vi "After Launch Init.vi"(8 "error in (no error)":errorcluster, 11 "LS218 in":refnum<class "LS218.lvclass">) -> (0 "error out":errorcluster, 3 "LS218 out":refnum<class "LS218.lvclass">)   [LabVIEW 2013, in "LS218.lvlib" / "LS218.lvclass"]
doc: "Use <b>Pre Launch init.vi</b> method for sanity checks that are supposed to prevent the actor from launching if they fail. Use <B>this</B> method instead to initialize this actor when it has been activated. A corresponding high priority message will become dispatched before the <B>Actor Core.vi</b> is called.\n\n<b>Derived classed should call the parent methode first</b> and their own initialization code after.\n\nRefer also to the ongoing discussion at https://decibel.ni.com/content/message/57394#57394."
uses:
  LS218.lvclass
  LS218 Messages/Read All Sensor Data Msg/Read All Sensor Data Msg.lvclass
  LS218.lvclass/LS218.ctl
  CSPP_Core/Classes/CS++ProcessVariables/PVConnection/PVConnection.lvclass
  CSPP_Core/Actors/CS++DeviceActor/CS++DeviceActor.lvclass
  <vilib>/ActorFramework/Actor/Actor.lvclass/Actor.ctl
  <vilib>/ActorFramework/Message Enqueuer/Message Enqueuer.lvclass/Message Enqueuer.ctl
  CSPP_Core/Actors/CS++DeviceActor/CS++DeviceActor.lvclass/CS++DeviceActor.ctl
  <vilib>/ActorFramework/Message Enqueuer/Init from Existing Queue.vi
  <vilib>/ActorFramework/Message Enqueuer/Enqueue.vi
  <vilib>/ActorFramework/Message Priority Queue/Priority Enqueue.vi
  <vilib>/ActorFramework/Message Enqueuer/Message Enqueuer.lvclass
  LS218 Messages/Write calibration curves to instruments Msg/Write calibration curves to instruments Msg.lvclass
  <vilib>/ActorFramework/Actor/Actor.lvclass
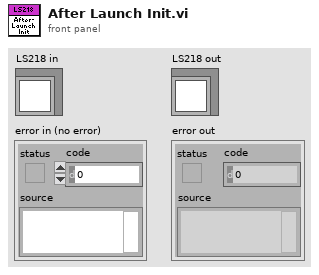
[diagram p1: front panel]
types:
  T1 = cluster{"Write Access":enum8{"Allowed", "Required", "None"}, "Read Access":enum8{"Allowed", "Required", "None"}}
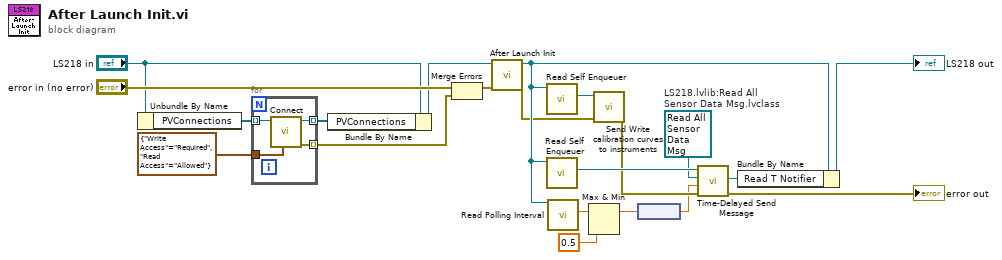
[diagram p0: block diagram]
diagram:
  w3 = refnum<class "Read All Sensor Data Msg.lvclass"> refnum  # LS218.lvlib:Read All Sensor Data Msg.lvclass
  n1 = Unbundle By Name("LS218 in") -> ("PVConnections"=w19:refnum<class "PVConnection.lvclass">[])
  n2 = for {
    tunnel: w19 -> [w25] mode=indexing
    tunnel: [w24] -> w18 mode=indexing
    tunnel: T1 {"Write Access"=enum."Required", "Read Access"=enum."Allowed"} ("Access") -> [w23]
    tunnel: [w22] -> w13 mode=indexing
    n3 = call-dynamic "Connect.vi"("Access (R/W allowed)"=w23, "PVConnection in"=w25) -> ("error out"=w22:errorcluster, "PVConnection out"=w24:refnum<class "PVConnection.lvclass">)  [unwired: 8 in]
  }
  n4 = Bundle By Name(cluster="LS218 in", "PVConnections"=w18) -> (w15:refnum<class "LS218.lvclass">)
  n5 = Merge Errors("error in (no error)", w13) -> (w14:errorcluster)
  n6 = call-parent "After Launch Init.vi"("error in (no error)"=w14, "CS++DeviceActor in"=w15) -> ("error out"=w1:errorcluster, "CS++DeviceActor out"=w2:refnum<class "LS218.lvclass">)  [unwired: 8 in]
  n7 = call <vilib>:"Read Self Enqueuer.vi"("Actor"=w2) -> ("Self Enqueuer"=w20:refnum<class "Message Enqueuer.lvclass">)  [unwired: 10 in]
  n8 = call <vilib>:"Read Self Enqueuer.vi"("Actor"=w2) -> ("Self Enqueuer"=w12:refnum<class "Message Enqueuer.lvclass">)  [unwired: 10 in]
  n9 = call "Read Polling Interval.vi"("CS++DeviceActor in"=w2) -> ("Polling Interval"=w7:dbl[unit])  [unwired: 8 in, 2 out]
  n10 = Max & Min(x=w7, y=dbl[unit] 0.5) -> (max(x,y)=w5:dbl[unit])  [unwired: 1 out]
  n11 = call "Send Write calibration curves to instruments.vi"("error in (no error)"=w1, "Message Enqueuer"=w20) -> ("error out"=w11:errorcluster)  [unwired: 8 in, 1 out]
  n12 = node(w5) -> (w6:dbl)
  n13 = call <vilib>:"Time-Delayed Send Message.vi"("error in (no error)"=w11, "Milliseconds To Wait"=w6, "Message"=w3, "Message Enqueuer"=w12) -> ("error out"=→"error out":errorcluster, "Delivery Notifier"=w8:refnum<notifier>)  [unwired: 6 in]
  n14 = Bundle By Name(cluster=w2, "Read T Notifier"=w8) -> (→"LS218 out":refnum<class "LS218.lvclass">)
